vi "FPGA Target.vi"() -> ()   [LabVIEW 2025]
uses:
  <vilib>/Platform/TimedLoop/XDataNode/wakeup.ctl
  <vilib>/Platform/TimedLoop/XDataNode/XDNodeRunTimeDep.lvlib
  <vilib>/Platform/TimedLoop/XDataNode/nitl_modes.ctl
  <vilib>/Platform/TimedLoop/XDataNode/timing_clust.ctl
  <vilib>/Platform/TimedLoop/XDataNode/XDataNode.xnode
  SubModules/Engine Simulation Toolkit FPGA IP/IP Source/APU/APU.lvlib
  <vilib>/rvi/DataTransferAndStorage/Container/XNode/niFpgaContainer.xnode
  Templates/FPGA Wizard Templates.lvlib
  <vilib>/rvi/interface/RandomDataEmulation/nirviRandomDataFpgaReadWriteTemplate.vi
  SubModules/Engine Simulation Toolkit FPGA IP/IP Source/Digital Pattern Generation/Digital Pattern Generation.lvlib
  SubModules/Engine Simulation Toolkit FPGA IP/IP Source/Directional Speed/Directional Speed.lvlib
  SubModules/FPGA Addon Speciality IO/Source/Speciality FPGA IO.lvlib
  SubModules/Engine Simulation Toolkit FPGA IP/IP Source/ECU Event/Timing/ECU Event Timing.lvlib
  SubModules/Engine Simulation Toolkit FPGA IP/IP Source/ECU Event/Timing/Measure Events (Non-40MHz).vi
  SubModules/Engine Simulation Toolkit FPGA IP/IP Source/ECU Event/Timing/Capture Settings.ctl
  SubModules/Engine Simulation Toolkit FPGA IP/IP Source/APU/Shared Settings.ctl
  SubModules/Engine Simulation Toolkit FPGA IP/IP Source/Version Token.ctl
  SubModules/Engine Simulation Toolkit FPGA IP/IP Source/Engine Simulation Toolkit.lvlib
  SubModules/Engine Simulation Toolkit FPGA IP/IP Source/APU/Settings.ctl
  SubModules/Engine Simulation Toolkit FPGA IP/IP Source/APU/Input.ctl
  SubModules/Engine Simulation Toolkit FPGA IP/IP Source/APU/Output.ctl
  SubModules/Engine Simulation Toolkit FPGA IP/IP Source/Digital Pattern Generation/Load Input.ctl
  SubModules/Engine Simulation Toolkit FPGA IP/IP Source/Directional Speed/Load Input.ctl
  SubModules/FPGA Addon Speciality IO/Source/Types/Static.Generate.Digital.Settings.ctl
  SubModules/FPGA Addon Speciality IO/Source/Types/PWM.Generate.Digital.Settings.ctl
  SubModules/FPGA Addon Speciality IO/Source/Types/PWM.Measure.Digital.Settings.ctl
  SubModules/FPGA Addon Speciality IO/Source/Types/PWM.Measure.Digital.Measurement.ctl
  SubModules/FPGA Addon Speciality IO/Source/Types/Static.Measure.Digital.Settings.ctl
  SubModules/FPGA Addon Speciality IO/Source/Types/Static.Measure.Digital.Measurement.ctl
  SubModules/Engine Simulation Toolkit FPGA IP/IP Source/Digital Pattern Generation/Settings.ctl
  SubModules/Engine Simulation Toolkit FPGA IP/IP Source/Digital Pattern Generation/Input.ctl
  SubModules/FPGA Addon Speciality IO/Source/Types/WSS.Generate.Digital.Settings.ctl
  SubModules/Engine Simulation Toolkit FPGA IP/IP Source/Directional Speed/Settings.ctl
  SubModules/Engine Simulation Toolkit FPGA IP/IP Source/Directional Speed/Input.ctl
  SubModules/Engine Simulation Toolkit FPGA IP/IP Source/ECU Event/Timing/Measure Settings.ctl
  SubModules/Engine Simulation Toolkit FPGA IP/IP Source/ECU Event/Timing/Measure Output.ctl
  SubModules/Engine Simulation Toolkit FPGA IP/IP Source/ECU Event/Timing/Capture Output.ctl
panel:
  out "capture.Cyl Inj 2.Event 4":T1
  out "capture.Cyl Inj 2.Event 3":T1
  out "capture.Cyl Inj 2.Event 2":T1
  out "capture.Cyl Inj 2.Event 1":T1
  out "status.Cyl Inj 2":T2
  in  "settings.Cyl Inj 2":T3
  out "capture.Cyl Inj 1.Event 4":T1
  out "capture.Cyl Inj 1.Event 3":T1
  out "capture.Cyl Inj 1.Event 2":T1
  out "capture.Cyl Inj 1.Event 1":T1
  out "status.Cyl Inj 1":T2
  in  "settings.Cyl Inj 1":T3
  out "PWM IN 2.Measure":T4
  in  "PWM IN 2.Settings":T5={"ACTIVE EDGE"=TRUE, "TIMEOUT"=40000000}
  out "PWM IN 1.Measure":T4
  in  "PWM IN 1.Settings":T5={"ACTIVE EDGE"=TRUE, "TIMEOUT"=40000000}
  out "Mod5.Monitor":bool[](array[boolean])
  out "Mod4.Monitor":bool[](array[boolean])
  in  "input.Crank":T6
  in  "settings.Crank":T7
  in  "input.Crank_Temp":T8
  in  "settings.Crank_Temp":T9
  in  "Front Driver WS.Settings":T10={"ACTIVE EDGE"=TRUE, "ACTIVE TICKS"=0, "INACTIVE TICKS"=0, "DATA"=0, "SENSOR TYPE"=0}
  in  "input.Exhaust CAM 1":T8
  in  "settings.Exhaust CAM 1":T9
  in  "input.Intake CAM 1":T8
  in  "settings.Intake CAM 1":T9
  in  "PWM Out 2.Settings":T11={"ACTIVE EDGE"=TRUE, "ACTIVE TICKS"=0, "INACTIVE TICKS"=0}
  in  "PWM Out 1.Settings":T11={"ACTIVE EDGE"=TRUE, "ACTIVE TICKS"=0, "INACTIVE TICKS"=0}
  out "State 35.Measure":T12
  in  "State 35.Settings":T13={"ACTIVE EDGE"=TRUE}
  out "State 34.Measure":T12
  in  "State 34.Settings":T13={"ACTIVE EDGE"=TRUE}
  out "State 33.Measure":T12
  in  "State 33.Settings":T13={"ACTIVE EDGE"=TRUE}
  out "State 32.Measure":T12
  in  "State 32.Settings":T13={"ACTIVE EDGE"=TRUE}
  out "State 31.Measure":T12
  in  "State 31.Settings":T13={"ACTIVE EDGE"=TRUE}
  out "State 30.Measure":T12
  in  "State 30.Settings":T13={"ACTIVE EDGE"=TRUE}
  out "State 29.Measure":T12
  in  "State 29.Settings":T13={"ACTIVE EDGE"=TRUE}
  out "State 28.Measure":T12
  in  "State 28.Settings":T13={"ACTIVE EDGE"=TRUE}
  out "State 27.Measure":T12
  in  "State 27.Settings":T13={"ACTIVE EDGE"=TRUE}
  out "State 26.Measure":T12
  in  "State 26.Settings":T13={"ACTIVE EDGE"=TRUE}
  out "State 25.Measure":T12
  in  "State 25.Settings":T13={"ACTIVE EDGE"=TRUE}
  out "State 24.Measure":T12
  in  "State 24.Settings":T13={"ACTIVE EDGE"=TRUE}
  out "State 23.Measure":T12
  in  "State 23.Settings":T13={"ACTIVE EDGE"=TRUE}
  out "State 22.Measure":T12
  in  "State 22.Settings":T13={"ACTIVE EDGE"=TRUE}
  out "State 21.Measure":T12
  in  "State 21.Settings":T13={"ACTIVE EDGE"=TRUE}
  out "State 20.Measure":T12
  in  "State 20.Settings":T13={"ACTIVE EDGE"=TRUE}
  out "State 19.Measure":T12
  in  "State 19.Settings":T13={"ACTIVE EDGE"=TRUE}
  out "State 18.Measure":T12
  in  "State 18.Settings":T13={"ACTIVE EDGE"=TRUE}
  out "State 17.Measure":T12
  in  "State 17.Settings":T13={"ACTIVE EDGE"=TRUE}
  out "State 16.Measure":T12
  in  "State 16.Settings":T13={"ACTIVE EDGE"=TRUE}
  out "State 15.Measure":T12
  in  "State 15.Settings":T13={"ACTIVE EDGE"=TRUE}
  out "State 14.Measure":T12
  in  "State 14.Settings":T13={"ACTIVE EDGE"=TRUE}
  out "State 13.Measure":T12
  in  "State 13.Settings":T13={"ACTIVE EDGE"=TRUE}
  out "State 12.Measure":T12
  in  "State 12.Settings":T13={"ACTIVE EDGE"=TRUE}
  out "State 11":bool
  out "State 10":bool
  out "State 9":bool
  out "State 8":bool
  out "State 7":bool
  out "State 6":bool
  out "State 5":bool
  out "State 4":bool
  out "Mod8.Monitor":bool[](array[boolean])
  out "State 3":bool
  out "State 2":bool
  out "State 1":bool
  out "State 0":bool
  out "PWM IN 6.Measure":T4
  in  "PWM IN 6.Settings":T5={"ACTIVE EDGE"=TRUE, "TIMEOUT"=40000000}
  out "PWM IN 5.Measure":T4
  in  "PWM IN 5.Settings":T5={"ACTIVE EDGE"=TRUE, "TIMEOUT"=40000000}
  out "PWM IN 4.Measure":T4
  in  "PWM IN 4.Settings":T5={"ACTIVE EDGE"=TRUE, "TIMEOUT"=40000000}
  out "PWM IN 3.Measure":T4
  in  "PWM IN 3.Settings":T5={"ACTIVE EDGE"=TRUE, "TIMEOUT"=40000000}
  out "Mod7.Monitor":bool[](array[boolean])
  out "Mod6.Monitor":bool[](array[boolean])
  in  "Output 4":bool
  in  "Output 3":bool
  in  "Output 2":bool
  in  "Output 1":bool
  in  "Output 0":bool
  in  "PWM Out 27.Settings":T11={"ACTIVE EDGE"=TRUE, "ACTIVE TICKS"=0, "INACTIVE TICKS"=0}
  in  "PWM Out 26.Settings":T11={"ACTIVE EDGE"=TRUE, "ACTIVE TICKS"=0, "INACTIVE TICKS"=0}
  in  "PWM Out 25.Settings":T11={"ACTIVE EDGE"=TRUE, "ACTIVE TICKS"=0, "INACTIVE TICKS"=0}
  in  "PWM Out 24.Settings":T11={"ACTIVE EDGE"=TRUE, "ACTIVE TICKS"=0, "INACTIVE TICKS"=0}
  in  "PWM Out 23.Settings":T11={"ACTIVE EDGE"=TRUE, "ACTIVE TICKS"=0, "INACTIVE TICKS"=0}
  in  "PWM Out 22.Settings":T11={"ACTIVE EDGE"=TRUE, "ACTIVE TICKS"=0, "INACTIVE TICKS"=0}
  in  "PWM Out 21.Settings":T11={"ACTIVE EDGE"=TRUE, "ACTIVE TICKS"=0, "INACTIVE TICKS"=0}
  in  "PWM Out 20.Settings":T11={"ACTIVE EDGE"=TRUE, "ACTIVE TICKS"=0, "INACTIVE TICKS"=0}
  in  "PWM Out 19.Settings":T11={"ACTIVE EDGE"=TRUE, "ACTIVE TICKS"=0, "INACTIVE TICKS"=0}
  in  "PWM Out 18.Settings":T11={"ACTIVE EDGE"=TRUE, "ACTIVE TICKS"=0, "INACTIVE TICKS"=0}
  in  "PWM Out 17.Settings":T11={"ACTIVE EDGE"=TRUE, "ACTIVE TICKS"=0, "INACTIVE TICKS"=0}
  in  "PWM Out 16.Settings":T11={"ACTIVE EDGE"=TRUE, "ACTIVE TICKS"=0, "INACTIVE TICKS"=0}
  in  "PWM Out 15.Settings":T11={"ACTIVE EDGE"=TRUE, "ACTIVE TICKS"=0, "INACTIVE TICKS"=0}
  in  "PWM Out 14.Settings":T11={"ACTIVE EDGE"=TRUE, "ACTIVE TICKS"=0, "INACTIVE TICKS"=0}
  in  "PWM Out 13.Settings":T11={"ACTIVE EDGE"=TRUE, "ACTIVE TICKS"=0, "INACTIVE TICKS"=0}
  in  "PWM Out 12.Settings":T11={"ACTIVE EDGE"=TRUE, "ACTIVE TICKS"=0, "INACTIVE TICKS"=0}
  in  "PWM Out 11.Settings":T11={"ACTIVE EDGE"=TRUE, "ACTIVE TICKS"=0, "INACTIVE TICKS"=0}
  in  "PWM Out 10.Settings":T11={"ACTIVE EDGE"=TRUE, "ACTIVE TICKS"=0, "INACTIVE TICKS"=0}
  in  "PWM Out 9.Settings":T11={"ACTIVE EDGE"=TRUE, "ACTIVE TICKS"=0, "INACTIVE TICKS"=0}
  in  "PWM Out 8.Settings":T11={"ACTIVE EDGE"=TRUE, "ACTIVE TICKS"=0, "INACTIVE TICKS"=0}
  in  "PWM Out 7.Settings":T11={"ACTIVE EDGE"=TRUE, "ACTIVE TICKS"=0, "INACTIVE TICKS"=0}
  in  "PWM Out 6.Settings":T11={"ACTIVE EDGE"=TRUE, "ACTIVE TICKS"=0, "INACTIVE TICKS"=0}
  in  "PWM Out 5.Settings":T11={"ACTIVE EDGE"=TRUE, "ACTIVE TICKS"=0, "INACTIVE TICKS"=0}
  in  "PWM Out 4.Settings":T11={"ACTIVE EDGE"=TRUE, "ACTIVE TICKS"=0, "INACTIVE TICKS"=0}
  in  "PWM Out 3.Settings":T11={"ACTIVE EDGE"=TRUE, "ACTIVE TICKS"=0, "INACTIVE TICKS"=0}
  in  "PWM Out 2.Settings":T11={"ACTIVE EDGE"=TRUE, "ACTIVE TICKS"=0, "INACTIVE TICKS"=0}
  in  "PWM Out 1.Settings":T11={"ACTIVE EDGE"=TRUE, "ACTIVE TICKS"=0, "INACTIVE TICKS"=0}
  out "Mod3.Monitor":bool[](array[boolean])
  in  "Power 15.Settings":T14={"ACTIVE EDGE"=TRUE, "OUTPUT"=FALSE}
  in  "Power 14.Settings":T14={"ACTIVE EDGE"=TRUE, "OUTPUT"=FALSE}
  in  "Power 13.Settings":T14={"ACTIVE EDGE"=TRUE, "OUTPUT"=FALSE}
  in  "Power 12.Settings":T14={"ACTIVE EDGE"=TRUE, "OUTPUT"=FALSE}
  in  "Power 11.Settings":T14={"ACTIVE EDGE"=TRUE, "OUTPUT"=FALSE}
  in  "Power 10.Settings":T14={"ACTIVE EDGE"=TRUE, "OUTPUT"=FALSE}
  in  "Power 9.Settings":T14={"ACTIVE EDGE"=TRUE, "OUTPUT"=FALSE}
  in  "Power 8.Settings":T14={"ACTIVE EDGE"=TRUE, "OUTPUT"=FALSE}
  out "Mod2.Monitor":bool[](array[boolean])
  in  "Power 7":bool
  in  "Power 6":bool
  in  "Power 5":bool
  in  "Power 4":bool
  out "Mod1.Monitor":bool[](array[boolean])
  in  "Power 3":bool
  in  "Power 2":bool
  in  "Power 1":bool
  in  "Power 0":bool
  in  "load input.Crank":T15
  in  "load input.Crank_Temp":T16
  in  "load input.Exhaust CAM 1":T16
  in  "load input.Intake CAM 1":T16
  out "Actual Analog Input Loop Period (usec)":u32
  out "Actual Analog Output Loop Period (usec)":u32
  out "Actual Digital Loop Period (usec)":u32
  out "Actual DMA Loop Period (usec)":u32
  in  "Analog Input Loop Timer (uSec)":u32=10
  out "output.apu 1":T17 caption="output"
  in  "input.apu 1":T18={"desired speed"=0.0, "reset"=TRUE} caption="input"
  in  "settings.apu 1":T19 caption="settings"
  in  "est.version":T20
  in  "shared settings.apu 1":T21 {"start" format="%#.15g"}
  in  "go.apu 1":bool
  in  "Digital Loop Timer (uSec)":u32=10
  in  "Analog Output Loop Timer (uSec)":u32=10
  in  "DMA.Enable":bool
  in  "DMA.MinimumSamples":u32=100000 caption="DMA Loop Timer (uSec)"
  out "DMA.Timeout":bool
  in  "DMA.Timeout.Reset":bool
  in  "DMA Loop Timer (uSec)":u32=10
types:
  T1 = typedef "Engine Simulation Toolkit.lvlib/ECU Event Timing.lvlib/Capture Output.ctl" = cluster{"Start":u16, "End":u16, "Duration (tics)":fxp<+,18,18>, "Event present":bool}
  T2 = typedef "Engine Simulation Toolkit.lvlib/ECU Event Timing.lvlib/Measure Output.ctl" = cluster{"stuck active":bool, "window all active":bool, "window orphan start":bool, "window orphan end":bool}
  T3 = typedef "Engine Simulation Toolkit.lvlib/ECU Event Timing.lvlib/Measure Settings.ctl" = cluster{"max":u16, "min":u16, "active high":bool, "wrap":bool}
  T4 = typedef "Speciality FPGA IO.lvlib/PWM.Measure.Digital.Measurement.ctl" = cluster{"ACTIVE TICKS":u32, "INACTIVE TICKS":u32, "ACQ TICKS":u32}
  T5 = typedef "Speciality FPGA IO.lvlib/PWM.Measure.Digital.Settings.ctl" = cluster{"ACTIVE EDGE":bool, "TIMEOUT":u32}
  T6 = typedef "Engine Simulation Toolkit.lvlib/Directional Speed.lvlib/Input.ctl" = cluster{"td (tics)":u16, "tf (tics)":u16, "tr (tics)":u16}
  T7 = typedef "Engine Simulation Toolkit.lvlib/Directional Speed.lvlib/Settings.ctl" = cluster{"Upper Value":u16, "Lower Value":u16, "Upper Index":fxp<+,10,10>, "Lower Index":fxp<+,10,10>, "Enabled":bool}
  T8 = typedef "Engine Simulation Toolkit.lvlib/Digital Pattern Generation.lvlib/Input.ctl" = cluster{"Offset":i16}
  T9 = typedef "Engine Simulation Toolkit.lvlib/Digital Pattern Generation.lvlib/Settings.ctl" = cluster{"edge 1":u16, "edge 2":u16, "cycle angle":bool, "enabled":bool, "first falling":bool, "fault":bool, "fault wrap":bool, "fault value":bool, "fault count":fxp<+,4,4>, "use fault count":bool}
  T10 = typedef "Speciality FPGA IO.lvlib/WSS.Generate.Digital.Settings.ctl" = cluster{"ACTIVE EDGE":bool, "ACTIVE TICKS":u32, "INACTIVE TICKS":u32, "DATA":u8, "SENSOR TYPE":u8}
  T11 = typedef "Speciality FPGA IO.lvlib/PWM.Generate.Digital.Settings.ctl" = cluster{"ACTIVE EDGE":bool, "ACTIVE TICKS":u32, "INACTIVE TICKS":u32}
  T12 = typedef "Speciality FPGA IO.lvlib/Static.Measure.Digital.Measurement.ctl" = cluster{"STATE":bool}
  T13 = typedef "Speciality FPGA IO.lvlib/Static.Measure.Digital.Settings.ctl" = cluster{"ACTIVE EDGE":bool}
  T14 = typedef "Speciality FPGA IO.lvlib/Static.Generate.Digital.Settings.ctl" = cluster{"ACTIVE EDGE":bool, "OUTPUT":bool}
  T15 = typedef "Engine Simulation Toolkit.lvlib/Directional Speed.lvlib/Load Input.ctl" = cluster{"address":fxp<+,10,10>, "done":bool, "angle":u16}
  T16 = typedef "Engine Simulation Toolkit.lvlib/Digital Pattern Generation.lvlib/Load Input.ctl" = cluster{"address":fxp<+,11,11>, "done":bool, "angle":u16}
  T17 = typedef "Engine Simulation Toolkit.lvlib/APU.lvlib/Output.ctl" = cluster{"crank":u16, "cycle":u16, "actual speed":fxp<+/-,23,2>}
  T18 = typedef "Engine Simulation Toolkit.lvlib/APU.lvlib/Input.ctl" = cluster{"desired speed":fxp<+/-,23,2>, "reset":bool}
  T19 = typedef "Engine Simulation Toolkit.lvlib/APU.lvlib/Settings.ctl" = cluster{"acceleration":fxp<+,18,-20>, "enable accel":bool}
  T20 = typedef "Engine Simulation Toolkit.lvlib/Version Token.ctl" = cluster{"1.4.0":bool}
  T21 = typedef "Engine Simulation Toolkit.lvlib/APU.lvlib/Shared Settings.ctl" = cluster{"start":fxp<+,17,17>, "stuck limit":fxp<+,18,18>}
  T22 = typedef "XDNodeRunTimeDep.lvlib/timing_clust.ctl" = cluster{"Expected End [f-1]":u64, "Actual End [f-1]":u64, "Finished Late? [f-1]":bool, "Expected End [i-1]":u64, "Actual End [i-1]":u64, "Finished Late? [i-1]":bool, "Expected Start [i]":u64, "Actual Start [i]":u64, "Expected Start [f]":u64, "Actual Start [f]":u64, "Source Name":string, "Structure Name":string, "Period":i64, "Deadline":i64, "Offset":i64, "Start":i64, "Priority":i32, "Timeout":i32, "Mode":T23, "Wakeup Reason":T24, "Error":errorcluster, "Source Type":string, "Secondary Source Type":string, "Global End Time":u64, "Global Start Time":u64, "Frame Duration":u64, "Iteration Duration":u64, "Assigned CPU":i32, "I/O Scan Engine Mode":u32}
  T23 = typedef "XDNodeRunTimeDep.lvlib/nitl_modes.ctl" = enum32{"No Change", "Process missed periods, maintain original phase", "Discard missed periods, maintain original phase", "Process missed periods, ignore original phase", "Discard missed periods, ignore original phase"}
  T24 = typedef "XDNodeRunTimeDep.lvlib/wakeup.ctl" = enum32{"Normal", "Aborted", "Asynchronous wakeup", "Timing source error", "Timed loop error", "Timeout"}
  T25 = typedef "Engine Simulation Toolkit.lvlib/ECU Event Timing.lvlib/Capture Settings.ctl" = u8
  T26 = cluster{"DI 0":refnum<k21>, "DI 1":refnum<k21>, "DI 2":refnum<k21>, "DI 3":refnum<k21>}
  T27 = cluster{"DO 0":refnum<k21>, "DO 1":refnum<k21>, "DO 2":refnum<k21>, "DO 3":refnum<k21>, "DO 4":refnum<k21>, "DO 5":refnum<k21>, "DO 6":refnum<k21>, "DO 7":refnum<k21>}
  T28 = cluster{"DI 0":refnum<k21>, "DI 1":refnum<k21>, "DI 2":refnum<k21>, "DI 3":refnum<k21>, "DI 4":refnum<k21>, "DI 5":refnum<k21>, "DI 6":refnum<k21>, "DI 7":refnum<k21>, "DI 8":refnum<k21>, "DI 9":refnum<k21>, "DI 10":refnum<k21>, "DI 11":refnum<k21>, "DI 12":refnum<k21>, "DI 13":refnum<k21>, "DI 14":refnum<k21>, "DI 15":refnum<k21>, "DI 16":refnum<k21>, "DI 17":refnum<k21>, "DI 18":refnum<k21>, "DI 19":refnum<k21>, "DI 20":refnum<k21>, "DI 21":refnum<k21>, "DI 22":refnum<k21>, "DI 23":refnum<k21>, "DI 24":refnum<k21>, "DI 25":refnum<k21>, "DI 26":refnum<k21>, "DI 27":refnum<k21>, "DI 28":refnum<k21>, "DI 29":refnum<k21>, "DI 30":refnum<k21>, "DI 31":refnum<k21>}
  T29 = cluster{"DI 0":refnum<k21>, "DI 1":refnum<k21>, "DI 2":refnum<k21>, "DI 3":refnum<k21>, "DI 4":refnum<k21>, "DI 5":refnum<k21>, "DI 6":refnum<k21>, "DI 7":refnum<k21>}
  T30 = cluster{"DO 0":refnum<k21>, "DO 1":refnum<k21>, "DO 2":refnum<k21>, "DO 3":refnum<k21>, "DO 4":refnum<k21>, "DO 5":refnum<k21>, "DO 6":refnum<k21>, "DO 7":refnum<k21>, "DO 8":refnum<k21>, "DO 9":refnum<k21>, "DO 10":refnum<k21>, "DO 11":refnum<k21>, "DO 12":refnum<k21>, "DO 13":refnum<k21>, "DO 14":refnum<k21>, "DO 15":refnum<k21>, "DO 16":refnum<k21>, "DO 17":refnum<k21>, "DO 18":refnum<k21>, "DO 19":refnum<k21>, "DO 20":refnum<k21>, "DO 21":refnum<k21>, "DO 22":refnum<k21>, "DO 23":refnum<k21>, "DO 24":refnum<k21>, "DO 25":refnum<k21>, "DO 26":refnum<k21>, "DO 27":refnum<k21>, "DO 28":refnum<k21>, "DO 29":refnum<k21>, "DO 30":refnum<k21>, "DO 31":refnum<k21>}
  T31 = cluster{"DO 0":refnum<k21>, "DO 1":refnum<k21>, "DO 2":refnum<k21>, "DO 3":refnum<k21>}
  T32 = typedef "Engine Simulation Toolkit.lvlib/Digital Pattern Generation.lvlib/Load Data.ctl" = cluster{"max address":fxp<+,11,11>, "memory":refnum<k21>}
  T33 = typedef "Engine Simulation Toolkit.lvlib/Directional Speed.lvlib/Load Data.ctl" = cluster{"max address":fxp<+,10,10>, "Memory":refnum<k21>}
  T34 = typedef "Engine Simulation Toolkit.lvlib/APU.lvlib/Register Bus.ctl" = cluster{"Speed":refnum<k21>, "Crank Angle":refnum<k21>, "Cycle Angle":refnum<k21>, "Crank Count":refnum<k21>, "Cycle Count":refnum<k21>, "1.25 MHz Counter":refnum<k21>, "Crank Rollover":refnum<k21>, "Cycle Rollover":refnum<k21>, "shared settings":T21}
  T35 = typedef "Engine Simulation Toolkit.lvlib/ECU Event Timing.lvlib/Measured Data.ctl" = cluster{"start":u16, "end":u16, "duration (tics)":fxp<+,18,18>, "window end":bool, "window begin":bool, "pulse end":bool, "pulse #":u8}
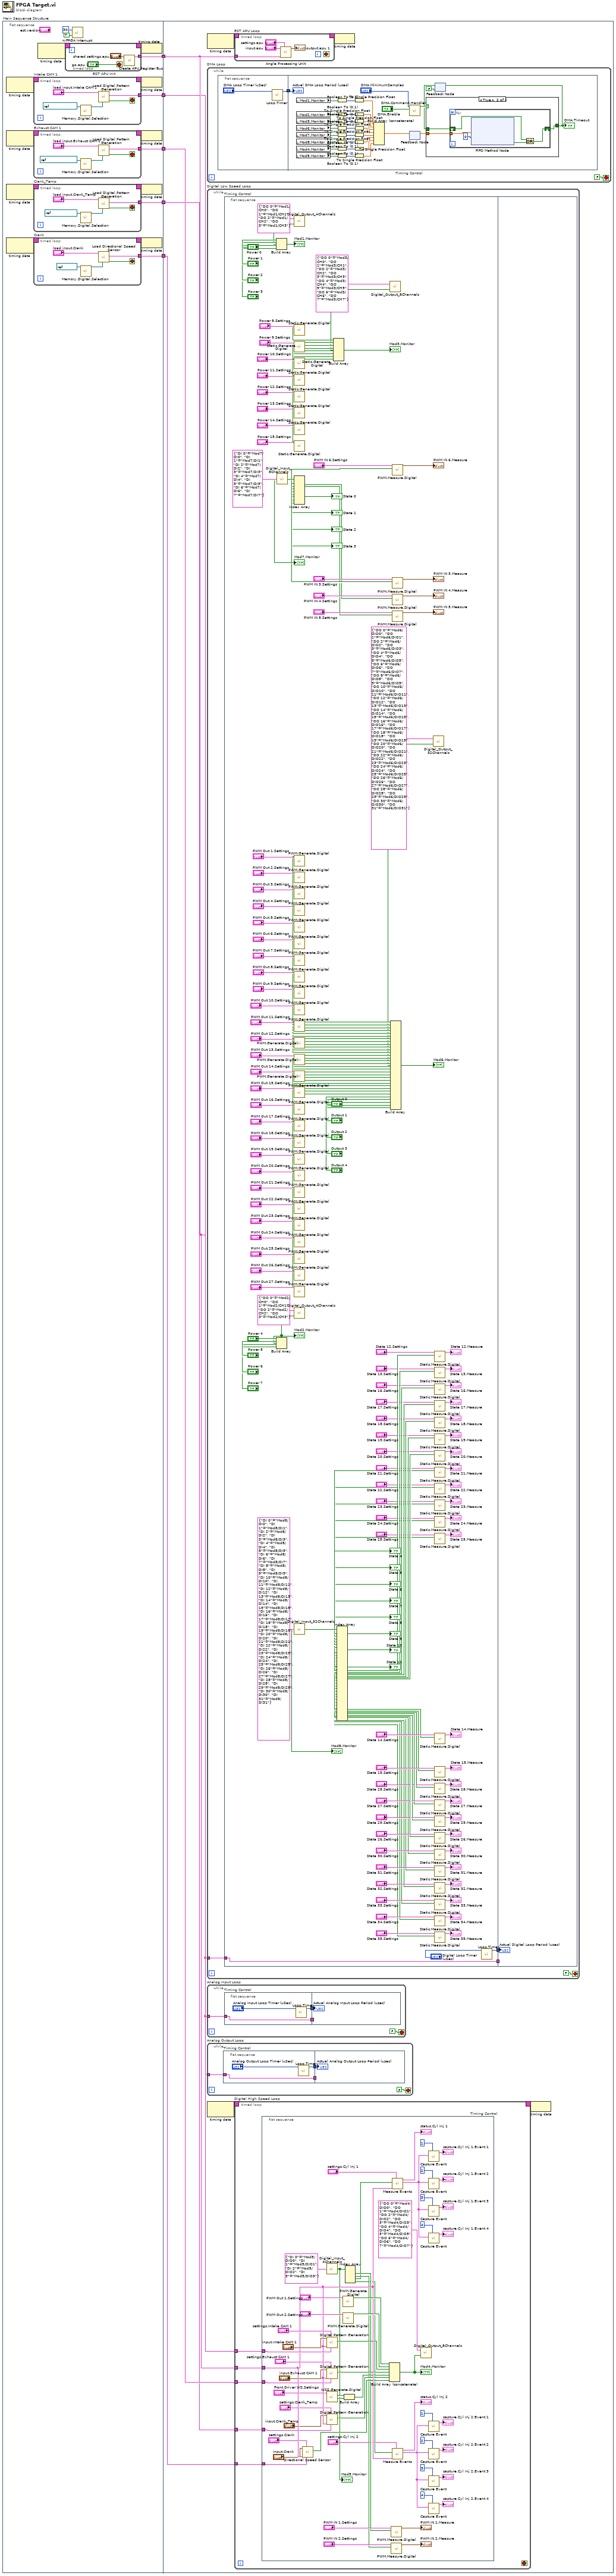
[diagram p0: block diagram]
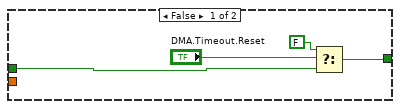
[diagram p2: hidden frame]
diagram:
  n1 = flat-sequence "Main Sequence Structure" {
    tunnel: [w18] -> w5
    tunnel: [w9] -> w4
    tunnel: [w8] -> w3
    tunnel: [w7] -> w2
    tunnel: [w6] -> w1
    tunnel: w5 -> [w70]
    tunnel: w4 -> [w69]
    tunnel: w3 -> [w68]
    tunnel: w2 -> [w67]
    tunnel: w1 -> [w66]
    frame #0 {
      n2 = node-c288() -> (w17:T22)  [unwired: 1 in]
      n3 = node-c288() -> (w15:T22)  [unwired: 1 in]
      n4 = node-c288() -> (w13:T22)  [unwired: 1 in]
      n5 = node-c288() -> (w11:T22)  [unwired: 1 in]
      n6 = timed-loop "Intake CAM 1" {
        timing: w17 -> [_]
        timing-out: [_] -> w16
        tunnel: [w50] -> w9
        stop <- w53 stop-if-true
        n7 = call "Memory.Digital.Selection.vi"("memory"=refnum<k21> "Intake CAM 1") -> ("memory"=w51:refnum<k21>)  [unwired: 10 in]
        n8 = call "Load Digital Pattern Generation.vi"("memory"=w51, "load input.<user name>"="load input.Intake CAM 1") -> ("done"=w53:bool, "load data"=w50:T32)  [unwired: 8 in]
      }
      n9 = timed-loop "Exhaust CAM 1" {
        timing: w15 -> [_]
        timing-out: [_] -> w14
        tunnel: [w41] -> w8
        stop <- w44 stop-if-true
        n10 = call "Memory.Digital.Selection.vi"("memory"=refnum<k21> "Exhaust CAM 1") -> ("memory"=w42:refnum<k21>)  [unwired: 10 in]
        n11 = call "Load Digital Pattern Generation.vi"("memory"=w42, "load input.<user name>"="load input.Exhaust CAM 1") -> ("done"=w44:bool, "load data"=w41:T32)  [unwired: 8 in]
      }
      n12 = timed-loop "Crank_Temp" {
        timing: w13 -> [_]
        timing-out: [_] -> w12
        tunnel: [w32] -> w7
        stop <- w35 stop-if-true
        n13 = call "Memory.Digital.Selection.vi"("memory"=refnum<k21> "Crank_Temp") -> ("memory"=w33:refnum<k21>)  [unwired: 10 in]
        n14 = call "Load Digital Pattern Generation.vi"("memory"=w33, "load input.<user name>"="load input.Crank_Temp") -> ("done"=w35:bool, "load data"=w32:T32)  [unwired: 8 in]
      }
      n15 = timed-loop "Crank" {
        timing: w11 -> [_]
        timing-out: [_] -> w10
        tunnel: [w23] -> w6
        stop <- w26 stop-if-true
        n16 = call "Memory.Digital.Selection.vi"("memory"=refnum<k21> "Crank") -> ("memory"=w24:refnum<k21>)  [unwired: 10 in]
        n17 = call "Load Directional Speed Sensor.vi"("Memory In"=w24, "load input.<user name>"="load input.Crank") -> ("done"=w26:bool, "load data"=w23:T33)  [unwired: 8 in]
      }
      n18 = node-c288() -> (w20:T22)  [unwired: 1 in]
      n19 = timed-loop "EST APU Init" {
        timing: w20 -> [_]
        timing-out: [_] -> w19
        tunnel: [w59] -> w18
        stop <- "go.apu 1" stop-if-true
        n20 = call "Create APU Register Bus.vi"("shared settings.<user name>"="shared settings.apu 1") -> ("register bus"=w59:T34)  [unwired: 10 in]
      }
      n21 = call <vilib>:"niFPGA Interrupt.vi"("Wait Until Cleared (F)"=TRUE, "IRQ Number (0)"=u8 30) -> ()  [unwired: 1 in]
      n22 = node-c288(w19) -> ()
      n23 = node-c288(w16) -> ()
      n24 = node-c288(w14) -> ()
      n25 = node-c288(w12) -> ()
      n26 = node-c288(w10) -> ()
    }
    frame #1 {
      # "FPGA Addon Code"
      n27 = node-c288 ("Input Node")() -> (w72:T22)  [unwired: 1 in]
      n28 = while "DMA Loop" {
        stop <- FALSE stop-if-true
        n29 = flat-sequence "Timing Control" {
          tunnel: [w153] -> w151
          tunnel: w151 -> [w179]
          frame #0 {
            n30 = call "Loop.Timer.vi"("Loop Timer (uSec)"="DMA Loop Timer (uSec)") -> ("Actual Loop Period (usec)"=w153:u32)  [unwired: 10 in]
          }
          frame #1 {
            n31 = local read "Mod1.Monitor"() -> (w178:bool[])
            n32 = local read "Mod2.Monitor"() -> (w176:bool[])
            n33 = local read "Mod3.Monitor"() -> (w174:bool[])
            n34 = local read "Mod6.Monitor"() -> (w172:bool[])
            n35 = local read "Mod7.Monitor"() -> (w170:bool[])
            n36 = local read "Mod8.Monitor"() -> (w168:bool[])
            n37 = local read "Mod4.Monitor"() -> (w166:bool[])
            n38 = local read "Mod5.Monitor"() -> (w164:bool[])
            n39 = Boolean To (0,1)(Boolean=w178) -> (0, 1=w177:i16[])
            n40 = Boolean To (0,1)(Boolean=w176) -> (0, 1=w175:i16[])
            n41 = Boolean To (0,1)(Boolean=w174) -> (0, 1=w173:i16[])
            n42 = Boolean To (0,1)(Boolean=w172) -> (0, 1=w171:i16[])
            n43 = Boolean To (0,1)(Boolean=w170) -> (0, 1=w169:i16[])
            n44 = Boolean To (0,1)(Boolean=w168) -> (0, 1=w167:i16[])
            n45 = Boolean To (0,1)(Boolean=w166) -> (0, 1=w165:i16[])
            n46 = Boolean To (0,1)(Boolean=w164) -> (0, 1=w163:i16[])
            n47 = To Single Precision Float(number=w177) -> (single precision float=w162:sgl[])
            n48 = To Single Precision Float(number=w175) -> (single precision float=w161:sgl[])
            n49 = To Single Precision Float(number=w173) -> (single precision float=w160:sgl[])
            n50 = To Single Precision Float(number=w171) -> (single precision float=w159:sgl[])
            n51 = To Single Precision Float(number=w169) -> (single precision float=w158:sgl[])
            n52 = To Single Precision Float(number=w167) -> (single precision float=w157:sgl[])
            n53 = To Single Precision Float(number=w165) -> (single precision float=w156:sgl[])
            n54 = To Single Precision Float(number=w163) -> (single precision float=w155:sgl[])
            n55 = Build Array (concatenate) "Build Array"(w162, w161, w160, w159, w158, w157, w156, w155) -> (w185:sgl[])
            n56 = call "DMA.Command.Handler.vi"("DMA.Enable"="DMA.Enable", "DMA.MinimumSamples"="DMA.MinimumSamples") -> ("Transfer"=w181:bool)  [unwired: 9 in]
            n57 = feedback #1() -> (w184:sgl[])  [unwired: 1 in]
            n58 = feedback-in #1(w185) -> ()
            n59 = feedback #2(FALSE ("t")) -> (w180:bool)
            n60 = case shown="True" w181 {
              tunnel: w184 -> [_ w194]
              tunnel: w180 -> [w189 w193]
              tunnel: [w188 w192] -> w183
              frame False {
                n61 = Select(t=FALSE, s="DMA.Timeout.Reset", f=w189) -> (s? t:f=w188:bool)
              }
              frame True {
                n62 = for {
                  shift-right: [w197] -> w192
                  shift-left: w193 -> [w196]
                  tunnel: w194 -> [w195] mode=indexing
                  n63 = xnode ("FIFO Method Node")("Element"=w195, "Timeout"=0) -> ("Timed Out?"=w198:bool)  [unwired: 1 in, 1 out]
                  n64 = Or(x=w196, y=w198) -> (x .or. y?=w197:bool)
                }
              }
            }
            "DMA.Timeout" <- w183
            n65 = feedback-in #2(w183) -> ()
            "Actual DMA Loop Period (usec)" <- w179
          }
        }
      }
      n66 = while "Digital Low Speed Loop" {
        tunnel: w70 -> [w218]
        stop <- FALSE stop-if-true
        n67 = flat-sequence "Timing Control" {
          tunnel: w218 -> [w413]
          tunnel: [w413] -> w217
          tunnel: [w411] -> w216
          tunnel: w217 -> [_]
          tunnel: w216 -> [w414]
          frame #0 {
            n68 = Build Array("Power 0", "Power 1", "Power 2", "Power 3") -> (w405:bool[])
            "Mod1.Monitor" <- w405
            n69 = Build Array("Power 4", "Power 5", "Power 6", "Power 7") -> (w399:bool[])
            "Mod2.Monitor" <- w399
            n70 = call "Digital_Input_8Channels.vi"("IO"=T29 {"DI 0"="Mod7/DI0", "DI 1"="Mod7/DI1", "DI 2"="Mod7/DI2", "DI 3"="Mod7/DI3", "DI 4"="Mod7/DI4", "DI 5"="Mod7/DI5", "DI 6"="Mod7/DI6", "DI 7"="Mod7/DI7"}) -> ("States"=w318:bool[])
            "Mod7.Monitor" <- w318
            n71 = call "Digital_Output_4Channels.vi"("States"=w405, "IO"=T31 {"DO 0"="Mod1/CH0", "DO 1"="Mod1/CH1", "DO 2"="Mod1/CH2", "DO 3"="Mod1/CH3"}) -> ()  [unwired: 1 in]
            n72 = call "Static.Generate.Digital.vi"("Settings"="Power 8.Settings") -> ("Output"=w390:bool)  [unwired: 10 in]
            n73 = call "Static.Generate.Digital.vi"("Settings"="Power 9.Settings") -> ("Output"=w389:bool)  [unwired: 10 in]
            n74 = call "Static.Generate.Digital.vi"("Settings"="Power 10.Settings") -> ("Output"=w388:bool)  [unwired: 10 in]
            n75 = call "Static.Generate.Digital.vi"("Settings"="Power 11.Settings") -> ("Output"=w387:bool)  [unwired: 10 in]
            n76 = call "Static.Generate.Digital.vi"("Settings"="Power 12.Settings") -> ("Output"=w386:bool)  [unwired: 10 in]
            n77 = call "Static.Generate.Digital.vi"("Settings"="Power 13.Settings") -> ("Output"=w385:bool)  [unwired: 10 in]
            n78 = call "Static.Generate.Digital.vi"("Settings"="Power 14.Settings") -> ("Output"=w384:bool)  [unwired: 10 in]
            n79 = call "Static.Generate.Digital.vi"("Settings"="Power 15.Settings") -> ("Output"=w383:bool)  [unwired: 10 in]
            n80 = Index Array(array=w318) -> (element #1=w316:bool, element #2=w313:bool, element #3=w310:bool, element #4=w307:bool, element #5=→"State 0":bool, element #6=→"State 1":bool, element #7=→"State 2":bool, element #8=→"State 3":bool)  [unwired: 8 in]
            n81 = call "PWM.Generate.Digital.vi"("Settings"="PWM Out 1.Settings") -> ("Output"=w353:bool)  [unwired: 10 in]
            n82 = call "PWM.Generate.Digital.vi"("Settings"="PWM Out 2.Settings") -> ("Output"=w352:bool)  [unwired: 10 in]
            n83 = call "PWM.Generate.Digital.vi"("Settings"="PWM Out 3.Settings") -> ("Output"=w351:bool)  [unwired: 10 in]
            n84 = call "PWM.Generate.Digital.vi"("Settings"="PWM Out 4.Settings") -> ("Output"=w350:bool)  [unwired: 10 in]
            n85 = call "PWM.Generate.Digital.vi"("Settings"="PWM Out 5.Settings") -> ("Output"=w349:bool)  [unwired: 10 in]
            n86 = call "PWM.Generate.Digital.vi"("Settings"="PWM Out 6.Settings") -> ("Output"=w348:bool)  [unwired: 10 in]
            n87 = call "PWM.Generate.Digital.vi"("Settings"="PWM Out 7.Settings") -> ("Output"=w347:bool)  [unwired: 10 in]
            n88 = call "PWM.Generate.Digital.vi"("Settings"="PWM Out 8.Settings") -> ("Output"=w346:bool)  [unwired: 10 in]
            n89 = call "PWM.Generate.Digital.vi"("Settings"="PWM Out 9.Settings") -> ("Output"=w345:bool)  [unwired: 10 in]
            n90 = call "PWM.Generate.Digital.vi"("Settings"="PWM Out 10.Settings") -> ("Output"=w344:bool)  [unwired: 10 in]
            n91 = call "PWM.Generate.Digital.vi"("Settings"="PWM Out 11.Settings") -> ("Output"=w343:bool)  [unwired: 10 in]
            n92 = call "PWM.Generate.Digital.vi"("Settings"="PWM Out 12.Settings") -> ("Output"=w342:bool)  [unwired: 10 in]
            n93 = call "PWM.Generate.Digital.vi"("Settings"="PWM Out 13.Settings") -> ("Output"=w341:bool)  [unwired: 10 in]
            n94 = call "PWM.Generate.Digital.vi"("Settings"="PWM Out 14.Settings") -> ("Output"=w340:bool)  [unwired: 10 in]
            n95 = call "PWM.Generate.Digital.vi"("Settings"="PWM Out 15.Settings") -> ("Output"=w339:bool)  [unwired: 10 in]
            n96 = call "PWM.Generate.Digital.vi"("Settings"="PWM Out 16.Settings") -> ("Output"=w338:bool)  [unwired: 10 in]
            n97 = call "PWM.Generate.Digital.vi"("Settings"="PWM Out 17.Settings") -> ("Output"=w337:bool)  [unwired: 10 in]
            n98 = call "PWM.Generate.Digital.vi"("Settings"="PWM Out 18.Settings") -> ("Output"=w336:bool)  [unwired: 10 in]
            n99 = call "PWM.Generate.Digital.vi"("Settings"="PWM Out 19.Settings") -> ("Output"=w335:bool)  [unwired: 10 in]
            n100 = call "PWM.Generate.Digital.vi"("Settings"="PWM Out 20.Settings") -> ("Output"=w334:bool)  [unwired: 10 in]
            n101 = call "PWM.Generate.Digital.vi"("Settings"="PWM Out 21.Settings") -> ("Output"=w333:bool)  [unwired: 10 in]
            n102 = call "PWM.Generate.Digital.vi"("Settings"="PWM Out 22.Settings") -> ("Output"=w332:bool)  [unwired: 10 in]
            n103 = call "PWM.Generate.Digital.vi"("Settings"="PWM Out 23.Settings") -> ("Output"=w331:bool)  [unwired: 10 in]
            n104 = call "PWM.Generate.Digital.vi"("Settings"="PWM Out 24.Settings") -> ("Output"=w330:bool)  [unwired: 10 in]
            n105 = call "PWM.Generate.Digital.vi"("Settings"="PWM Out 25.Settings") -> ("Output"=w329:bool)  [unwired: 10 in]
            n106 = call "PWM.Generate.Digital.vi"("Settings"="PWM Out 26.Settings") -> ("Output"=w328:bool)  [unwired: 10 in]
            n107 = call "PWM.Generate.Digital.vi"("Settings"="PWM Out 27.Settings") -> ("Output"=w327:bool)  [unwired: 10 in]
            n108 = call "Digital_Output_4Channels.vi"("States"=w399, "IO"=T31 {"DO 0"="Mod2/CH0", "DO 1"="Mod2/CH1", "DO 2"="Mod2/CH2", "DO 3"="Mod2/CH3"}) -> ()  [unwired: 1 in]
            n109 = call "Digital_Input_32Channels.vi"("IO"=T28 {"DI 0"="Mod8/DI0", "DI 1"="Mod8/DI1", "DI 2"="Mod8/DI2", "DI 3"="Mod8/DI3", "DI 4"="Mod8/DI4", "DI 5"="Mod8/DI5", "DI 6"="Mod8/DI6", "DI 7"="Mod8/DI7", "DI 8"="Mod8/DI8", "DI 9"="Mod8/DI9", "DI 10"="Mod8/DI10", "DI 11"="Mod8/DI11", "DI 12"="Mod8/DI12", "DI 13"="Mod8/DI13", "DI 14"="Mod8/DI14", "DI 15"="Mod8/DI15", "DI 16"="Mod8/DI16", "DI 17"="Mod8/DI17", "DI 18"="Mod8/DI18", "DI 19"="Mod8/DI19", "DI 20"="Mod8/DI20", "DI 21"="Mod8/DI21", "DI 22"="Mod8/DI22", "DI 23"="Mod8/DI23", "DI 24"="Mod8/DI24", "DI 25"="Mod8/DI25", "DI 26"="Mod8/DI26", "DI 27"="Mod8/DI27", "DI 28"="Mod8/DI28", "DI 29"="Mod8/DI29", "DI 30"="Mod8/DI30", "DI 31"="Mod8/DI31"}) -> ("States"=w300:bool[])
            "Mod8.Monitor" <- w300
            n110 = Build Array(w390, w389, w388, w387, w386, w385, w384, w383) -> (w381:bool[])
            "Mod3.Monitor" <- w381
            n111 = Index Array(array=w300) -> (element #1=→"State 4":bool, element #2=→"State 5":bool, element #3=→"State 6":bool, element #4=→"State 7":bool, element #5=→"State 8":bool, element #6=→"State 9":bool, element #7=→"State 10":bool, element #8=→"State 11":bool, element #9=w290:bool, element #10=w287:bool, element #11=w284:bool, element #12=w281:bool, element #13=w278:bool, element #14=w275:bool, element #15=w272:bool, element #16=w269:bool, element #17=w266:bool, element #18=w263:bool, element #19=w260:bool, element #20=w257:bool, element #21=w254:bool, element #22=w251:bool, element #23=w248:bool, element #24=w245:bool, element #25=w242:bool, element #26=w239:bool, element #27=w236:bool, element #28=w233:bool, element #29=w230:bool, element #30=w227:bool, element #31=w224:bool, element #32=w221:bool)  [unwired: 32 in]
            n112 = call "Digital_Output_8Channels.vi"("States"=w381, "IO"=T27 {"DO 0"="Mod3/CH0", "DO 1"="Mod3/CH1", "DO 2"="Mod3/CH2", "DO 3"="Mod3/CH3", "DO 4"="Mod3/CH4", "DO 5"="Mod3/CH5", "DO 6"="Mod3/CH6", "DO 7"="Mod3/CH7"}) -> ()  [unwired: 1 in]
            n113 = Build Array(w353, w352, w351, w350, w349, w348, w347, w346, w345, w344, w343, w342, w341, w340, w339, w338, w337, w336, w335, w334, w333, w332, w331, w330, w329, w328, w327, "Output 0", "Output 1", "Output 2", "Output 3", "Output 4") -> (w320:bool[])
            "Mod6.Monitor" <- w320
            n114 = call "PWM.Measure.Digital.vi"("State"=w307, "Settings"="PWM IN 6.Settings") -> ("Measurement"=→"PWM IN 6.Measure":T4)  [unwired: 8 in, 1 out]
            n115 = call "PWM.Measure.Digital.vi"("State"=w316, "Settings"="PWM IN 3.Settings") -> ("Measurement"=→"PWM IN 3.Measure":T4)  [unwired: 8 in, 1 out]
            n116 = call "PWM.Measure.Digital.vi"("State"=w313, "Settings"="PWM IN 4.Settings") -> ("Measurement"=→"PWM IN 4.Measure":T4)  [unwired: 8 in, 1 out]
            n117 = call "PWM.Measure.Digital.vi"("State"=w310, "Settings"="PWM IN 5.Settings") -> ("Measurement"=→"PWM IN 5.Measure":T4)  [unwired: 8 in, 1 out]
            n118 = call "Digital_Output_32Channels.vi"("States"=w320, "IO"=T30 {"DO 0"="Mod6/DIO0", "DO 1"="Mod6/DIO1", "DO 2"="Mod6/DIO2", "DO 3"="Mod6/DIO3", "DO 4"="Mod6/DIO4", "DO 5"="Mod6/DIO5", "DO 6"="Mod6/DIO6", "DO 7"="Mod6/DIO7", "DO 8"="Mod6/DIO8", "DO 9"="Mod6/DIO9", "DO 10"="Mod6/DIO10", "DO 11"="Mod6/DIO11", "DO 12"="Mod6/DIO12", "DO 13"="Mod6/DIO13", "DO 14"="Mod6/DIO14", "DO 15"="Mod6/DIO15", "DO 16"="Mod6/DIO16", "DO 17"="Mod6/DIO17", "DO 18"="Mod6/DIO18", "DO 19"="Mod6/DIO19", "DO 20"="Mod6/DIO20", "DO 21"="Mod6/DIO21", "DO 22"="Mod6/DIO22", "DO 23"="Mod6/DIO23", "DO 24"="Mod6/DIO24", "DO 25"="Mod6/DIO25", "DO 26"="Mod6/DIO26", "DO 27"="Mod6/DIO27", "DO 28"="Mod6/DIO28", "DO 29"="Mod6/DIO29", "DO 30"="Mod6/DIO30", "DO 31"="Mod6/DIO31"}) -> ()  [unwired: 1 in]
            n119 = call "Static.Measure.Digital.vi"("State"=w290, "Settings"="State 12.Settings") -> ("Measurement"=→"State 12.Measure":T12)  [unwired: 9 in]
            n120 = call "Static.Measure.Digital.vi"("State"=w287, "Settings"="State 13.Settings") -> ("Measurement"=→"State 13.Measure":T12)  [unwired: 9 in]
            n121 = call "Static.Measure.Digital.vi"("State"=w278, "Settings"="State 16.Settings") -> ("Measurement"=→"State 16.Measure":T12)  [unwired: 9 in]
            n122 = call "Static.Measure.Digital.vi"("State"=w275, "Settings"="State 17.Settings") -> ("Measurement"=→"State 17.Measure":T12)  [unwired: 9 in]
            n123 = call "Static.Measure.Digital.vi"("State"=w272, "Settings"="State 18.Settings") -> ("Measurement"=→"State 18.Measure":T12)  [unwired: 9 in]
            n124 = call "Static.Measure.Digital.vi"("State"=w269, "Settings"="State 19.Settings") -> ("Measurement"=→"State 19.Measure":T12)  [unwired: 9 in]
            n125 = call "Static.Measure.Digital.vi"("State"=w266, "Settings"="State 20.Settings") -> ("Measurement"=→"State 20.Measure":T12)  [unwired: 9 in]
            n126 = call "Static.Measure.Digital.vi"("State"=w263, "Settings"="State 21.Settings") -> ("Measurement"=→"State 21.Measure":T12)  [unwired: 9 in]
            n127 = call "Static.Measure.Digital.vi"("State"=w260, "Settings"="State 22.Settings") -> ("Measurement"=→"State 22.Measure":T12)  [unwired: 9 in]
            n128 = call "Static.Measure.Digital.vi"("State"=w257, "Settings"="State 23.Settings") -> ("Measurement"=→"State 23.Measure":T12)  [unwired: 9 in]
            n129 = call "Static.Measure.Digital.vi"("State"=w254, "Settings"="State 24.Settings") -> ("Measurement"=→"State 24.Measure":T12)  [unwired: 9 in]
            n130 = call "Static.Measure.Digital.vi"("State"=w251, "Settings"="State 25.Settings") -> ("Measurement"=→"State 25.Measure":T12)  [unwired: 9 in]
            n131 = call "Static.Measure.Digital.vi"("State"=w284, "Settings"="State 14.Settings") -> ("Measurement"=→"State 14.Measure":T12)  [unwired: 9 in]
            n132 = call "Static.Measure.Digital.vi"("State"=w281, "Settings"="State 15.Settings") -> ("Measurement"=→"State 15.Measure":T12)  [unwired: 9 in]
            n133 = call "Static.Measure.Digital.vi"("State"=w242, "Settings"="State 28.Settings") -> ("Measurement"=→"State 28.Measure":T12)  [unwired: 9 in]
            n134 = call "Static.Measure.Digital.vi"("State"=w245, "Settings"="State 27.Settings") -> ("Measurement"=→"State 27.Measure":T12)  [unwired: 9 in]
            n135 = call "Static.Measure.Digital.vi"("State"=w239, "Settings"="State 29.Settings") -> ("Measurement"=→"State 29.Measure":T12)  [unwired: 9 in]
            n136 = call "Static.Measure.Digital.vi"("State"=w248, "Settings"="State 26.Settings") -> ("Measurement"=→"State 26.Measure":T12)  [unwired: 9 in]
            n137 = call "Static.Measure.Digital.vi"("State"=w236, "Settings"="State 30.Settings") -> ("Measurement"=→"State 30.Measure":T12)  [unwired: 9 in]
            n138 = call "Static.Measure.Digital.vi"("State"=w233, "Settings"="State 31.Settings") -> ("Measurement"=→"State 31.Measure":T12)  [unwired: 9 in]
            n139 = call "Static.Measure.Digital.vi"("State"=w230, "Settings"="State 32.Settings") -> ("Measurement"=→"State 32.Measure":T12)  [unwired: 9 in]
            n140 = call "Static.Measure.Digital.vi"("State"=w227, "Settings"="State 33.Settings") -> ("Measurement"=→"State 33.Measure":T12)  [unwired: 9 in]
            n141 = call "Static.Measure.Digital.vi"("State"=w224, "Settings"="State 34.Settings") -> ("Measurement"=→"State 34.Measure":T12)  [unwired: 9 in]
            n142 = call "Static.Measure.Digital.vi"("State"=w221, "Settings"="State 35.Settings") -> ("Measurement"=→"State 35.Measure":T12)  [unwired: 9 in]
            n143 = call "Loop.Timer.vi"("Loop Timer (uSec)"="Digital Loop Timer (uSec)") -> ("Actual Loop Period (usec)"=w411:u32)  [unwired: 10 in]
          }
          frame #1 {
            "Actual Digital Loop Period (usec)" <- w414
          }
        }
      }
      n144 = while "Analog Input Loop" {
        tunnel: w70 -> [w210]
        stop <- FALSE stop-if-true
        n145 = flat-sequence "Timing Control" {
          tunnel: w210 -> [w214]
          tunnel: [w214] -> w209
          tunnel: [w212] -> w208
          tunnel: w209 -> [_]
          tunnel: w208 -> [w215]
          frame #0 {
            n146 = call "Loop.Timer.vi"("Loop Timer (uSec)"="Analog Input Loop Timer (uSec)") -> ("Actual Loop Period (usec)"=w212:u32)  [unwired: 10 in]
          }
          frame #1 {
            "Actual Analog Input Loop Period (usec)" <- w215
          }
        }
      }
      n147 = while "Analog Output Loop" {
        tunnel: w70 -> [w202]
        stop <- FALSE stop-if-true
        n148 = flat-sequence "Timing Control" {
          tunnel: w202 -> [w206]
          tunnel: [w206] -> w201
          tunnel: [w204] -> w200
          tunnel: w201 -> [_]
          tunnel: w200 -> [w207]
          frame #0 {
            n149 = call "Loop.Timer.vi"("Loop Timer (uSec)"="Analog Output Loop Timer (uSec)") -> ("Actual Loop Period (usec)"=w204:u32)  [unwired: 10 in]
          }
          frame #1 {
            "Actual Analog Output Loop Period (usec)" <- w207
          }
        }
      }
      n150 = node-c288() -> (w74:T22)  [unwired: 1 in]
      n151 = timed-loop "EST APU Loop" {
        timing: w72 -> [_]
        timing-out: [_] -> w71
        tunnel: w70 -> [w75]
        stop <- _ stop-if-true
        n152 = call "Angle Processing Unit.vi"("settings.<user name>"="settings.apu 1", "register bus"=w75, "input.<user name>"="input.apu 1") -> ("output.<user name>"=→"output.apu 1":T17)  [unwired: 8 in]
      }
      n153 = timed-loop "Digital High Speed Loop" {
        timing: w74 -> [_]
        timing-out: [_] -> w73
        tunnel: w70 -> [w87]
        tunnel: w69 -> [w86]
        tunnel: w68 -> [w85]
        tunnel: w67 -> [w84]
        tunnel: w66 -> [w83]
        stop <- _ stop-if-true
        n154 = flat-sequence "Timing Control" {
          tunnel: w87 -> [w141]
          tunnel: w86 -> [w142]
          tunnel: w85 -> [w138]
          tunnel: w84 -> [w132]
          tunnel: w83 -> [w129]
          frame #0 {
            n155 = call "Directional Speed Sensor.vi"("load data"=w129, "settings.<user name>"="settings.Crank", "register bus"=w141, "input.<user name>"="input.Crank") -> ("digial output"=w122:bool)  [unwired: 7 in]
            n156 = call "Digital_Input_4Channels.vi"("IO"=T26 {"DI 0"="Mod5/DIO0", "DI 1"="Mod5/DIO1", "DI 2"="Mod5/DIO2", "DI 3"="Mod5/DIO3"}) -> ("States"=w118:bool[])
            "Mod5.Monitor" <- w118
            n157 = call "Digital Pattern Generation.vi"("load data"=w142, "settings.<user name>"="settings.Intake CAM 1", "register bus"=w141, "input.<user name>"="input.Intake CAM 1") -> ("digial output"=w126:bool)  [unwired: 7 in]
            n158 = call "Digital Pattern Generation.vi"("load data"=w138, "settings.<user name>"="settings.Exhaust CAM 1", "register bus"=w141, "input.<user name>"="input.Exhaust CAM 1") -> ("digial output"=w125:bool)  [unwired: 7 in]
            n159 = call "WSS.Generate.Digital.vi"("Settings"="Front Driver WS.Settings") -> ("Bit1"=w135:bool, "Bit0"=w136:bool)  [unwired: 8 in, 1 out]
            n160 = call "Digital Pattern Generation.vi"("load data"=w132, "settings.<user name>"="settings.Crank_Temp", "register bus"=w141, "input.<user name>"="input.Crank_Temp") -> ("digial output"=w123:bool)  [unwired: 7 in]
            n161 = call "PWM.Generate.Digital.vi"("Settings"="PWM Out 1.Settings") -> ("Output"=w128:bool)  [unwired: 10 in]
            n162 = call "PWM.Generate.Digital.vi"("Settings"="PWM Out 2.Settings") -> ("Output"=w127:bool)  [unwired: 10 in]
            n163 = Build Array(w136, w135) -> (w124:bool[])
            n164 = Index Array(array=w118) -> (element #1=w116:bool, element #2=w113:bool, element #3=w110:bool, element #4=w98:bool)  [unwired: 4 in]
            n165 = Build Array (concatenate)(w128, w127, w126, w125, w124, w123, w122) -> (w120:bool[])
            "Mod4.Monitor" <- w120
            n166 = call "PWM.Measure.Digital.vi"("State"=w116, "Settings"="PWM IN 1.Settings") -> ("Measurement"=→"PWM IN 1.Measure":T4)  [unwired: 8 in, 1 out]
            n167 = call "PWM.Measure.Digital.vi"("State"=w113, "Settings"="PWM IN 2.Settings") -> ("Measurement"=→"PWM IN 2.Measure":T4)  [unwired: 8 in, 1 out]
            n168 = call-poly "Measure Events.vi"("settings.<user name>"="settings.Cyl Inj 1", "register bus"=w141, "event"=w110) -> ("measured data"=w107:T35, "status.<user name>"=→"status.Cyl Inj 1":T2)  [unwired: 7 in]
            n169 = call-poly "Measure Events.vi"("settings.<user name>"="settings.Cyl Inj 2", "register bus"=w141, "event"=w98) -> ("measured data"=w95:T35, "status.<user name>"=→"status.Cyl Inj 2":T2)  [unwired: 7 in]
            n170 = call "Digital_Output_8Channels.vi"("States"=w120, "IO"=T27 {"DO 0"="Mod4/DIO0", "DO 1"="Mod4/DIO1", "DO 2"="Mod4/DIO2", "DO 3"="Mod4/DIO3", "DO 4"="Mod4/DIO4", "DO 5"="Mod4/DIO5", "DO 6"="Mod4/DIO6", "DO 7"="Mod4/DIO7"}) -> ()  [unwired: 1 in]
            n171 = call "Capture Event.vi"("event # to capture"=T25 1, "measured data"=w107) -> ("capture.<user name>"=→"capture.Cyl Inj 1.Event 1":T1)  [unwired: 9 in]
            n172 = call "Capture Event.vi"("event # to capture"=T25 2, "measured data"=w107) -> ("capture.<user name>"=→"capture.Cyl Inj 1.Event 2":T1)  [unwired: 9 in]
            n173 = call "Capture Event.vi"("event # to capture"=T25 3, "measured data"=w107) -> ("capture.<user name>"=→"capture.Cyl Inj 1.Event 3":T1)  [unwired: 9 in]
            n174 = call "Capture Event.vi"("event # to capture"=T25 4, "measured data"=w107) -> ("capture.<user name>"=→"capture.Cyl Inj 1.Event 4":T1)  [unwired: 9 in]
            n175 = call "Capture Event.vi"("event # to capture"=T25 1, "measured data"=w95) -> ("capture.<user name>"=→"capture.Cyl Inj 2.Event 1":T1)  [unwired: 9 in]
            n176 = call "Capture Event.vi"("event # to capture"=T25 2, "measured data"=w95) -> ("capture.<user name>"=→"capture.Cyl Inj 2.Event 2":T1)  [unwired: 9 in]
            n177 = call "Capture Event.vi"("event # to capture"=T25 3, "measured data"=w95) -> ("capture.<user name>"=→"capture.Cyl Inj 2.Event 3":T1)  [unwired: 9 in]
            n178 = call "Capture Event.vi"("event # to capture"=T25 4, "measured data"=w95) -> ("capture.<user name>"=→"capture.Cyl Inj 2.Event 4":T1)  [unwired: 9 in]
          }
        }
      }
      n179 = node-c288 ("Output Node")(w71) -> ()
      n180 = node-c288 ("Output Node")(w73) -> ()
    }
  }
